vi "Expt4_MT PSK Transceiver_Student_lab.vi"(0 "Message Symbols":i32=1000, 5 "Eb/N0, dB":dbl(slide)=40.0 scale=0.0..80.0, 7 "TX Filter":T1(ring)=enum."Root Raised Cos", 9 "Reset":bool=TRUE, 14 "?":T2(tab)=enum."Constellation (RX output)") -> (3 "PSK System Parameters":T5={"samples per symbol (16)"=4, "symbol map"=[0.7071067811865476+0.7071067811865475i, -0.7071067811865475+0.7071067811865476i, 0.7071067811865474-0.7071067811865477i, -0.7071067811865477-0.7071067811865475i], "differential PSK"=enum."disable", "PSK type"=0} {"PSK type" items=["normal", "shifted", "offset"]; "symbol map" format="%.3f"}, 4 "Output Complex Waveform":cluster{"t0":dbl, "dt":dbl, "Values":cdb[]} {"Values" format="%.3f"; "dt" format="%^.2e"; "t0" format="%.4f"}, 6 "Transmitted  Bits":i8[](array[numeric]), 8 "Received Bits":i8[](array[numeric]), 10 "Bit Error Rate":dbl format="%.4e", 13 "Last Sync Found Index":dbl format="%.4f", 15 "Error Out":errorcluster)   [LabVIEW 2020]
doc: "This example demonstrates generation and analysis of PSK modulated signals. You can specify transmit filter parameters, Eb/No, and frequency offset. This example demonstrates programming techniques for resetting the transmitter in cases where the receiver (demodulator) lock is lost. You can see the results of the demodulation on an eye-diagram plot, and perform measurements such as bit error rate."
uses:
  <vilib>/addons/Modulation/niDMT.lvlib
  <vilib>/addons/Modulation/Digital/General/MT Format Eye Diagram (complex).vi
  <vilib>/addons/Modulation/niAMT.lvlib
  <vilib>/addons/Modulation/Digital/Demodulation/MT EbN0 Calculation(ASK).vi
  <vilib>/addons/Modulation/Digital/Support/Controls/PSK System Parameters.ctl
panel:
  out "Estimated Eb/N0(dB)":dbl
  out "Frequency Offset, Hz":dbl=0.0014081098665354938 format="%.2f"
  in  "Frequency Offset, Hz":dbl(slide) scale=-1000.0..1000.0
  in  "Symbol Rate":dbl=100000.0 step=1000.0 format="%.2p"
  in  "M-PSK":enum16{"2", "4", "8", "16", "32", "64"}(ring)=enum."4"
  out "Modulation Error Ratio, dB":dbl format="%.2f"
  out "BER Trigger Found":bool
  in  "Stop":bool
  out "TX Symbols":T3(graph)={{"1/x"=0.0, 1e-05, [], 1}, []}
  out "FFT Magnitude Spectrum":cluster{dbl, dbl, dbl[]}(graph)={-199899.99999999997, 99.99999999999999, []}
  out "Constellation graph":T4(graph)
  out "RX Symbols":T3(graph)={{"1/x"=0.0, 1e-05, [], 1}, []}
  in  "autoscale":bool
  out "Constellation Graph":T4(graph)
  in  "Display I/Q":enum16{"I", "Q"}(ring)=enum."Q"
  out "Eye Diagram":cluster{"t0":dbl, "dt":dbl, "Y":dbl[]}[](graph)
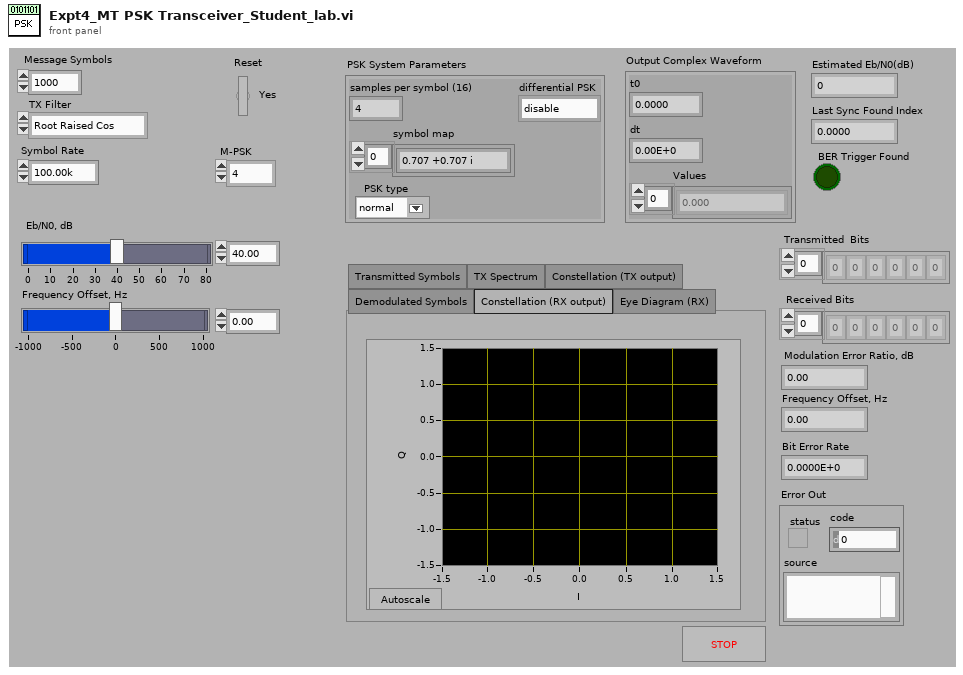
[diagram p1: front panel]
types:
  T1 = enum16{"none", "Raised Cosine", "Root Raised Cos", "Gaussian"}
  T2 = enum32{"Transmitted Symbols", "TX Spectrum", "Constellation (TX output)", "Demodulated Symbols", "Constellation (RX output)", "Eye Diagram (RX)"}
  T3 = cluster{cluster{"1/x":dbl, dbl, i8[], i32}, i32[][]}
  T4 = cluster{"Decimated Array":dbl[], "Decimated Array":dbl[]}[]
  T5 = typedef "niDMT.lvlib/PSK System Parameters.ctl" = cluster{"samples per symbol (16)":i32, "symbol map":cdb[], "differential PSK":enum16{"disable", "enable"}, "PSK type":u16}
  T6 = cluster{"expected sync location (symbols)":i32, "sync sequence":cdb[], "sync location uncertainty (symbols)":i32, "sync indent (symbols)":i32}
  T7 = cluster{"TX Filter":enum16{"none", "Raised Cosine", "Root Raised Cos", "Gaussian"}, "filter parameter":dbl, "filter length":i32}
  T8 = cluster{"M-PSK (4)":i32, "differential PSK":enum16{"disable", "enable"}, "PSK type":u16}
  T9 = cluster{"# Guard Bits":i32, "# Sync Bits":i32, "# Message Bits":i32, "PN sequence order":i32}
  T10 = cluster{"Output Bit Stream":i8[], " # bits per symbol":i32, "Sync (Bits)":i8[], "Sync (Symbols)":cdb[], "pulse shaping filter coefficients":dbl[], "matched filter coefficients":dbl[], "PSK system parameters":T5}
  T11 = typedef "niAMT.lvlib/Complex Data Waveform.ctl" = cluster{"t0":dbl, "dt":dbl, "Y":cdb[]}
  T12 = cluster{"constellation":dbl[], "oversampled data":dbl[]}[]
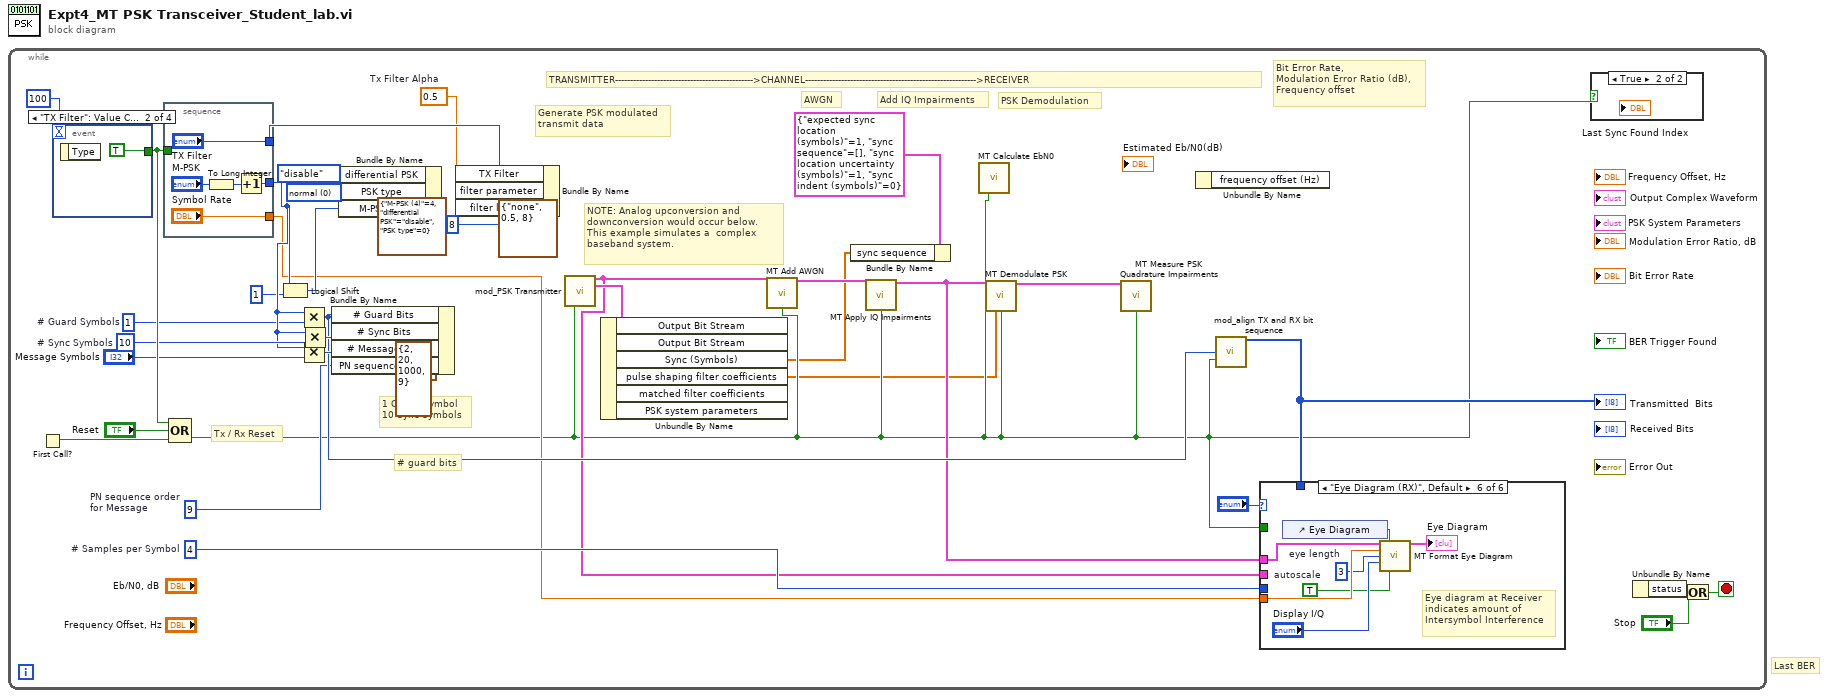
[diagram p0: block diagram]
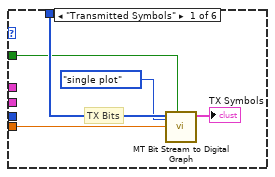
[diagram p2: hidden frame]
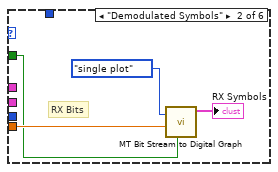
[diagram p3: hidden frame]
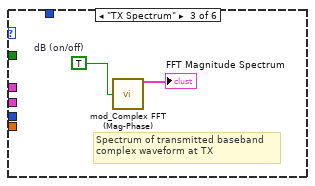
[diagram p4: hidden frame]
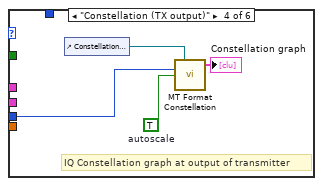
[diagram p5: hidden frame]
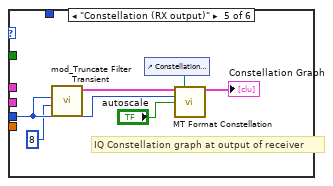
[diagram p6: hidden frame]
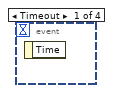
[diagram p8: hidden frame]
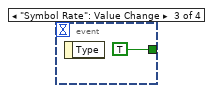
[diagram p9: hidden frame]
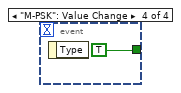
[diagram p10: hidden frame]
diagram:
  # "Last BER"
  n1 = while {
    stop <- w20 stop-if-true
    w10 = 9  # PN sequence order for Message
    w12 = 0.5  # Tx Filter Alpha
    w14 = u16 0 items=["normal", "shifted", "offset"] ("PSK type")
    w27 = 4  # # Samples per Symbol
    w30 = 10  # # Sync Symbols
    w23 = 1  # # Guard Symbols
    # "Bit Error Rate,\nModulation Error Ratio (dB),\nFrequency offset"
    # "Tx / Rx Reset"
    # "1 Guard Symbol\n10 Sync Symbols"
    # "# guard bits"
    # "Generate PSK modulated\ntransmit data"
    # "PSK Demodulation"
    # "Add IQ Impairments"
    # "AWGN"
    # "TRANSMITTER---------------------------------------------->CHANNEL--------------------------------------------------------->RECEIVER"
    # "NOTE: Analog upconversion and\ndownconversion would occur below.\nThis example simulates a  complex \nbaseband system."
    n2 = First Call?() -> (First Call?: T/F=w35:bool)
    n3 = event shown="[1] \"TX Filter\": Value Change" {
      selector: _ -> [_ _ _ _]
      dyn-events: _ -> [_ _ _ _]
      timeout: 100 -> [_ _ _ _]
      tunnel: [_ TRUE TRUE TRUE] -> w32
      event Timeout {
        n4 = event-data() -> ()  [unwired: 1 in, 1 out]
      }
      event "TX Filter": Value Change {
        n5 = event-data() -> ()  [unwired: 1 in, 1 out]
      }
      event "Symbol Rate": Value Change {
        n6 = event-data() -> ()  [unwired: 1 in, 1 out]
      }
      event "M-PSK": Value Change {
        n7 = event-data() -> ()  [unwired: 1 in, 1 out]
      }
    }
    n8 = stacked-sequence {
      tunnel: w32 -> [_]
      tunnel: ["TX Filter"] -> w28
      tunnel: [w39] -> w24
      tunnel: ["Symbol Rate"] -> w17
      frame #0 {
        n9 = To Long Integer(number="M-PSK") -> (32bit integer=w41:i32)
        n10 = Increment(x=w41) -> (x+1=w39:i32)
      }
    }
    n11 = Compound Arithmetic op=OR(w32, "Reset", w35) -> (w3:bool)
    n12 = Logical Shift(y=w24, x=1) -> (x << y=w19:i32)
    n13 = Multiply(x=w24, y=w23) -> (x*y=w22:i32)
    n14 = Multiply(x=w24, y="Message Symbols") -> (x*y=w25:i32)
    n15 = Multiply(x=w24, y=w30) -> (x*y=w29:i32)
    n16 = Bundle By Name(cluster=T9 {"# Guard Bits"=2, "# Sync Bits"=20, "# Message Bits"=1000, "PN sequence order"=9} ("Message"), "# Guard Bits"=w22, "# Sync Bits"=w29, "# Message Bits"=w25, "PN sequence order"=w10) -> ()  [unwired: 1 out]
    n17 = Bundle By Name(cluster=T8 {"M-PSK (4)"=4, "differential PSK"=enum."disable", "PSK type"=0} ("PSK"), "differential PSK"=enum16{"disable", "enable"}."disable", "PSK type"=w14, "M-PSK (4)"=w19) -> ()  [unwired: 1 out]
    n18 = Bundle By Name(cluster=T7 {"TX Filter"=enum."none", "filter parameter"=0.5, "filter length"=8} ("System Filter"), "TX Filter"=w28, "filter parameter"=w12, "filter length"=8) -> ()  [unwired: 1 out]
    n19 = call <vilib>:"mod_PSK Transmitter.vi"("Reset?"=w3) -> ("Output Complex Waveform"=w4:cluster{"t0":dbl, "dt":dbl, "Y":cdb[]}, "Signal Description"=w8:T10)  [unwired: 12 in, 1 out]
    n20 = Unbundle By Name(w8) -> ("Sync (Symbols)"=w2:cdb[], "pulse shaping filter coefficients"=w1:dbl[])  [unwired: 4 out]
    n21 = call <vilib>:"MT Add AWGN.vi"("input complex waveform"=w4, "reset? (T)"=w3) -> ("output complex waveform"=w7:T11)  [unwired: 11 in, 2 out]
    n22 = Bundle By Name(cluster=T6 {"expected sync location (symbols)"=1, "sync sequence"=[], "sync location uncertainty (symbols)"=1, "sync indent (symbols)"=0} ("synchronization parameters"), "sync sequence"=w2) -> ()  [unwired: 1 out]
    n23 = call <vilib>:"MT Apply IQ Impairments.vi"("input complex waveform"=w7, "reset? (T)"=w3) -> ("output complex waveform"=w5:T11)  [unwired: 12 in, 1 out]
    n24 = call-poly <vilib>:"MT Calculate EbN0.vi"("reset? (T)"=w3) -> ()  [unwired: 12 in, 3 out]
    n25 = call <vilib>:"MT Demodulate PSK.vi"("input complex waveform"=w5, "pulse shaping filter coefficients"=w1, "reset? (T)"=w3) -> ("recovered complex waveform"=w6:T11)  [unwired: 8 in, 4 out]
    n26 = call <vilib>:"MT Measure PSK Quadrature Impairments.vi"("recovered complex waveform"=w6, "reset? (T)"=w3) -> ()  [unwired: 6 in, 8 out]
    n27 = Unbundle By Name() -> ()  [unwired: 1 in, 1 out]
    n28 = call <vilib>:"mod_align TX and RX bit sequence.vi"("# Bits removed"=w22, "Reset"=w3) -> ("Aligned array"=w21:i8[])  [unwired: 13 in]
    "Transmitted  Bits" <- w21
    n29 = case shown="\"Eye Diagram (RX)\", Default" "?" {
      tunnel: w17 -> [w47 w51 _ _ _ w70]
      tunnel: w27 -> [_ _ _ w54 w60 _]
      tunnel: w21 -> [w46 _ _ _ _ _]
      tunnel: w3 -> [w45 w48 _ _ _ _]
      tunnel: w5 -> [_ _ _ _ _ w64]
      tunnel: w4 -> [_ _ _ _ _ _]
      frame "Transmitted Symbols" {
        # "TX Bits"
        n30 = call <vilib>:"MT Bit Stream to Digital Graph.vi"("Reset (F)"=w45, "Format"=enum16{"single plot", "plot per bit"}."single plot", "Symbol Rate (Hz)"=w47, "Bit Stream"=w46) -> ("Digital Waveform Graph"=→"TX Symbols":T3)  [unwired: 7 in]
      }
      frame "Demodulated Symbols" {
        # "RX Bits"
        n31 = call <vilib>:"MT Bit Stream to Digital Graph.vi"("Reset (F)"=w48, "Format"=enum16{"single plot", "plot per bit"}."single plot", "Symbol Rate (Hz)"=w51) -> ("Digital Waveform Graph"=→"RX Symbols":T3)  [unwired: 8 in]
      }
      frame "TX Spectrum" {
        w52 = TRUE  # dB (on/off)
        # "Spectrum of transmitted baseband\ncomplex waveform at TX"
        n32 = call <vilib>:"mod_Complex FFT (Mag-Phase).vi"("dB (on/off)"=w52) -> ("Magnitude"=→"FFT Magnitude Spectrum":cluster{"f0":dbl, "df":dbl, "Y":dbl[]})  [unwired: 13 in, 1 out]
      }
      frame "Constellation (TX output)" {
        w57 = TRUE  # autoscale
        # "IQ Constellation graph at output of transmitter"
        n33 = control-ref of="Constellation graph"() -> (w55:refnum<vi>)
        n34 = call <vilib>:"MT Format Constellation.vi"("constellation reference"=w55, "samples per symbol"=w54, "autoscale"=w57) -> ("constellation graph"=→"Constellation graph":T12)  [unwired: 11 in, 1 out]
      }
      frame "Constellation (RX output)" {
        # "IQ Constellation graph at output of receiver"
        n35 = call <vilib>:"mod_Truncate Filter Transient.vi"("filter length (sym)"=8, "samples/symbol"=w60) -> ("output complex waveform"=w61:T11)  [unwired: 9 in]
        n36 = control-ref of="Constellation Graph"() -> (w62:refnum<vi>)
        n37 = call <vilib>:"MT Format Constellation.vi"("waveform"=w61, "constellation reference"=w62, "samples per symbol"=w60, "autoscale"="autoscale") -> ("constellation graph"=→"Constellation Graph":T12)  [unwired: 10 in, 1 out]
      }
      frame "Eye Diagram (RX)", Default {
        w67 = TRUE  # autoscale
        w69 = 3  # eye length
        # "Eye diagram at Receiver\nindicates amount of\nIntersymbol Interference"
        n38 = control-ref of="Eye Diagram"() -> (w65:refnum<vi>)
        n39 = call-poly <vilib>:"MT Format Eye Diagram.vi"("waveform"=w64, "eye diagram reference"=w65, "symbol rate (Hz)"=w70, "eye length"=w69, "I/Q (I)"="Display I/Q", "autoscale"=w67) -> ("eye diagram"=→"Eye Diagram":cluster{"t0":dbl, "dt":dbl, "Y":dbl[]}[])  [unwired: 8 in, 1 out]
      }
    }
    n40 = case shown="True" w3 {
      frame False {
      }
      frame True {
      }
    }
    n41 = Unbundle By Name() -> ()  [unwired: 1 in, 1 out]
    n42 = Or(y="Stop") -> (x .or. y?=w20:bool)  [unwired: 1 in]
  }
